vi "startDio64.vi"(8 "error in (no error)":errorcluster, 11 "AtomChipHWC in":refnum<class "AtomChipHWC.lvclass">) -> (0 "error out":errorcluster, 3 "AtomChipHWC out":refnum<class "AtomChipHWC.lvclass">)   [LabVIEW 2009, in "Hardware.lvlib" / "HWControllers.lvlib" / "AtomChipHWC.lvclass"]
doc: "Start the DIO64 timing card"
uses:
  AtomChipHWC.lvclass
  AtomChipHWC.lvclass/AtomChipHWC.ctl
  Channels/Digital/DigitalOutput.lvclass
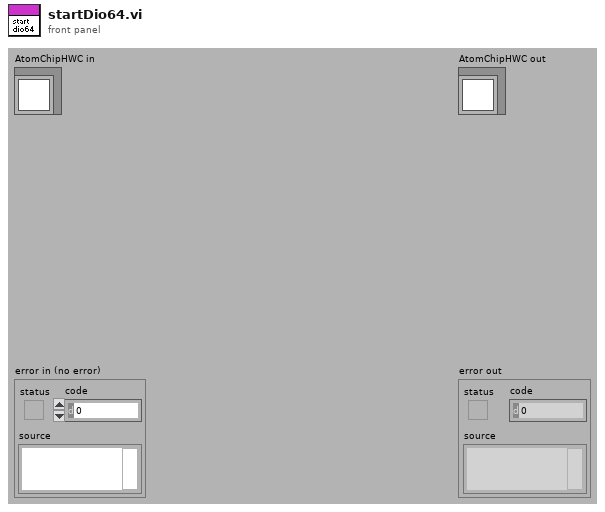
[diagram p1: front panel]
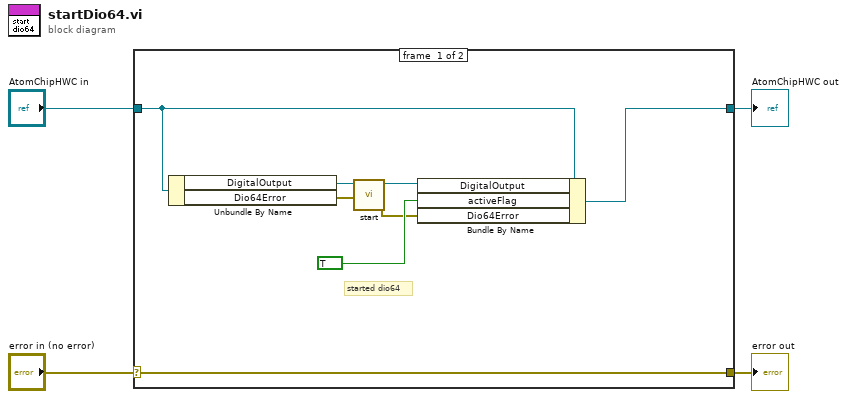
[diagram p0: block diagram]
diagram:
  n1 = case shown="No Error" "error in (no error)" {
    selector: "error in (no error)" -> [w5 w14]
    tunnel: [w5 w14] -> w3
    tunnel: [w9 w13] -> w1
    tunnel: "AtomChipHWC in" -> [w10 w13]
    frame #0 {
      # "started dio64"
      n2 = Unbundle By Name(w10) -> ("DigitalOutput"=w12:refnum<class "DigitalOutput.lvclass">, "Dio64Error"=w8:errorcluster)
      n3 = call-dynamic "start.vi"("error in (no error)"=w8, "DigitalOutput in"=w12) -> ("error out"=w6:errorcluster, "DigitalOutput out"=w11:refnum<class "DigitalOutput.lvclass">)  [unwired: 8 in]
      n4 = Bundle By Name(cluster=w10, "DigitalOutput"=w11, "activeFlag"=TRUE, "Dio64Error"=w6) -> (w9:refnum<class "AtomChipHWC.lvclass">)
    }
    frame #1 {
    }
  }
  "error out" <- w3
  "AtomChipHWC out" <- w1
